vi "Begin.vi"(8 "error in":errorcluster) -> (0 "error out":errorcluster)   [LabVIEW 2023]
doc: "Called before other user functions, this VI is expected to open initial I/O refnums, load in file data, and do all program initialization. Notice that the <B>error out</B> terminal is simply used for data flow. Wiring it to other structures or subVIs ensures that this VI runs first."
uses:
  <vilib>/Rock Robotics/WPI/DriverStation/WPI_DriverStationRobotMode2.ctl
  <vilib>/Rock Robotics/WPI/Joystick/WPI_JoystickDeviceEnum.ctl
  <vilib>/Rock Robotics/WPI/SafetyOutput/WPI_SafetyOutputConfigMenu.ctl
  <vilib>/Rock Robotics/WPI/RobotDrive/WPI_RobotDriveDevRef.ctl
  <vilib>/Rock Robotics/WPI/MotorControl/WPI_MotorControlDeviceRef.ctl
  <vilib>/Rock Robotics/WPI/MotorControl/WPI_MotorControlType.ctl
  <vilib>/Rock Robotics/SystemInterfaces/DIO/FPGA_DIOPWMChannel.ctl
  <vilib>/Rock Robotics/WPI/PWM/WPI_PWMDeadband.ctl
  <vilib>/Rock Robotics/SystemInterfaces/DIO/FPGA_DIOChannel.ctl
  <vilib>/Rock Robotics/WPI/ThirdParty/REV Robotics/REVLib/Typedef/Spark MAX Motor Type.ctl
  <vilib>/Rock Robotics/WPI/ThirdParty/REV Robotics/REVLib/Typedef/Spark MAX Idle Mode.ctl
  Robot Global Data.vi
  <vilib>/Rock Robotics/Network Tables/NT Write String Array.vi
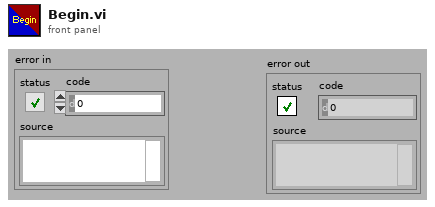
[diagram p1: front panel]
types:
  T1 = typedef "WPI_RobotDriveDevRef.ctl" = cluster{"DevStatus":errorcluster, "Motors[]":T2[], "Square Inputs":bool, "Max Output":dbl}
  T2 = typedef "WPI_MotorControlDeviceRef.ctl" = cluster{"DeviceStatus":errorcluster, "Type":T3, "PWM":cluster{"PWM Channel":T4, "DeadBand":T5}, "CAN":cluster{"Device Number":u8, "SetOutput VI Ref":variant, "GetOutput VI Ref":variant, "Enable VI Ref":variant, "Disable VI Ref":variant, "Data":variant}, "Invert":bool, "DIO PWM":cluster{"PWM \"Enable\" Channel":T4, "DIOChannel":T6, "PWM Rate":dbl}}
  T3 = typedef "WPI_MotorControlType.ctl" = enum16{"PWM", "CAN", "DIO PWM"}
  T4 = typedef "FPGA_DIOPWMChannel.ctl" = enum8{"PWM 0", "PWM 1", "PWM 2", "PWM 3", "PWM 4", "PWM 5", "PWM 6", "PWM 7", "PWM 8", "PWM 9", "PWM MXP 0", "PWM MXP 1", "PWM MXP 2", "PWM MXP 3", "PWM MXP 4", "PWM MXP 5", "PWM MXP 6", "PWM MXP 7", "PWM MXP 8", "PWM MXP 9", "Invalid"}
  T5 = typedef "WPI_PWMDeadband.ctl" = cluster{"Name":string, "maxPositivePwm":i32, "minPositivePwm":i32, "centerPwm":i32, "maxNegativePwm":i32, "minNegativePwm":i32, "angularRange":u16}
  T6 = typedef "FPGA_DIOChannel.ctl" = enum8{"DIO 0", "DIO 1", "DIO 2", "DIO 3", "DIO 4", "DIO 5", "DIO 6", "DIO 7", "DIO 8", "DIO 9", "DIO MXP 0", "DIO MXP 1", "DIO MXP 2", "DIO MXP 3", "DIO MXP 4", "DIO MXP 5", "DIO MXP 6", "DIO MXP 7", "DIO MXP 8", "DIO MXP 9", "DIO MXP 10", "DIO MXP 11", "DIO MXP 12", "DIO MXP 13", "DIO MXP 14", "DIO MXP 15", "SPI Port CS1", "SPI Port CS2", "SPI Port CS3", "SPI Port MISO", "SPI Port MOSI", "Invalid"}
  T7 = typedef "WPI_SafetyOutputConfigMenu.ctl" = enum16{"Enable", "Disable"}
  T8 = typedef "WPI_JoystickDeviceEnum.ctl" = enum16{"USB 0", "USB 1", "USB 2", "USB 3", "USB 4", "USB 5"}
  T9 = typedef "WPI_DriverStationRobotMode2.ctl" = enum16{"Autonomous Disabled", "Autonomous Enabled", "Teleop Disabled", "Teleop Enabled", "Disconnected", "Finish", "Test Disabled", "Test Enabled", "Emergency Stopped"}
  T10 = typedef "Spark MAX Idle Mode.ctl" = enum16{"Coast", "Brake"}
  T11 = typedef "Spark MAX Motor Type.ctl" = enum16{"Brushed", "Brushless"}
  T12 = typedef "WPI_JoystickDevRef.ctl" = cluster{"Device":T8}
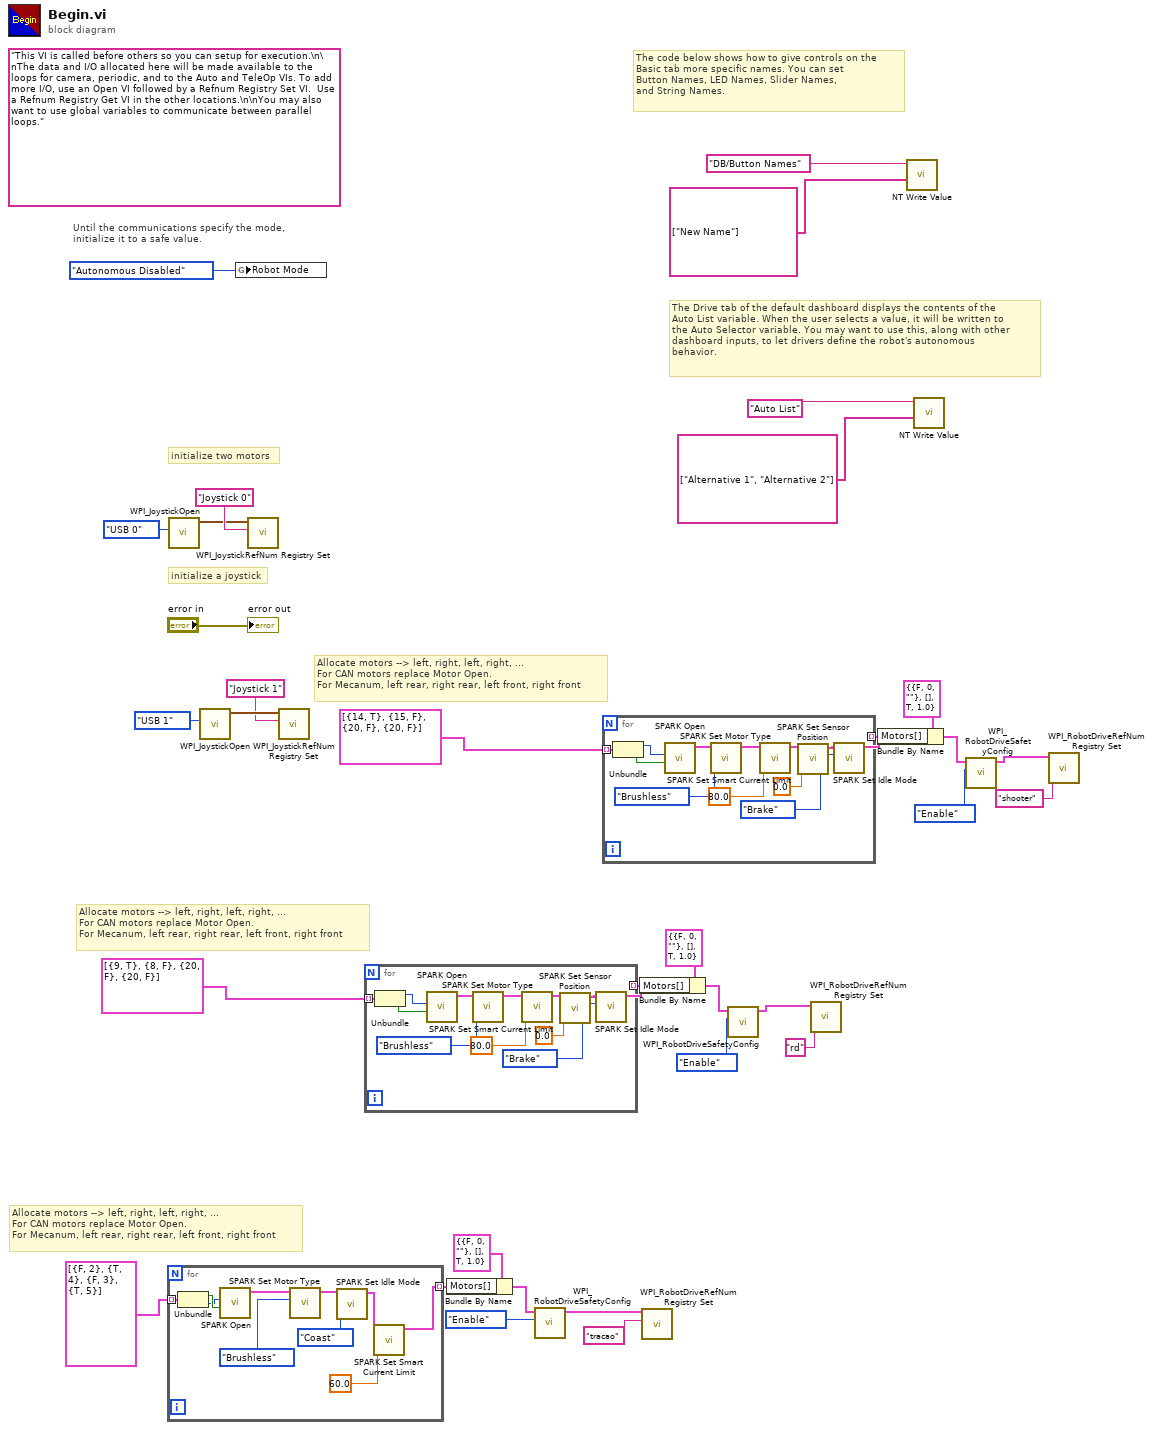
[diagram p0: block diagram]
diagram:
  (unwired) "This VI is called before others so you can setup for execution.\n\nThe data and I/O allocated here will be made available to the loops for camera, periodic, and to the Auto and TeleOp VIs. To add more I/O, use an Open VI followed by a Refnum Registry Set VI.  Use a Refnum Registry Get VI in the other locations.\n\nYou may also want to use global variables to communicate between parallel loops."
  # "Allocate motors --> left, right, left, right, ... \nFor CAN motors replace Motor Open.\nFor Mecanum, left rear, right rear, left front, right front"
  # "Allocate motors --> left, right, left, right, ... \nFor CAN motors replace Motor Open.\nFor Mecanum, left rear, right rear, left front, right front"
  # "Allocate motors --> left, right, left, right, ... \nFor CAN motors replace Motor Open.\nFor Mecanum, left rear, right rear, left front, right front"
  # "The Drive tab of the default dashboard displays the contents of the\nAuto List variable. When the user selects a value, it will be written to\nthe Auto Selector variable. You may want to use this, along with other\ndashboard inputs, to let drivers define the robot's autonomous\nbehavior."
  # "The code below shows how to give controls on the\nBasic tab more specific names. You can set\nButton Names, LED Names, Slider Names,\nand String Names."
  # "initialize a joystick"
  # "Until the communications specify the mode,\ninitialize it to a safe value."
  # "initialize two motors"
  n1 = for {
    tunnel: cluster{"Inverted":bool, "Motor Address":i32}[] [{"Inverted"=FALSE, "Motor Address"=2}, {"Inverted"=TRUE, "Motor Address"=4}, {"Inverted"=FALSE, "Motor Address"=3}, {"Inverted"=TRUE, "Motor Address"=5}] ("Array") -> [w43] mode=indexing
    tunnel: [w35] -> w10 mode=indexing
    n2 = Unbundle(w43) -> ("Inverted"=w42:bool, "Motor Address"=w41:i32)
    n3 = call <vilib>:"SPARK Open.vi"("Invert"=w42, "Device Number"=w41) -> ("MotorControlDeviceRef"=w40:T2)  [unwired: 8 in, 1 out]
    n4 = call <vilib>:"SPARK Set Motor Type.vi"("Motor Type"=Spark_MAX_Motor_Type."Brushless", "MotorControlDevRef"=w40) -> ("MotorControlDeviceRef"=w38:T2)  [unwired: 8 in, 1 out]
    n5 = call <vilib>:"SPARK Set Idle Mode.vi"("Idle Mode"=Spark_MAX_Idle_Mode."Coast", "MotorControlDeviceRef in"=w38) -> ("MotorControlDeviceRef out"=w36:T2)  [unwired: 8 in, 1 out]
    n6 = call <vilib>:"SPARK Set Smart Current Limit.vi"("Primay Current Limit (80A)"=60.0, "MotorControlDeviceRef in"=w36) -> ("MotorControlDeviceRef out"=w35:T2)  [unwired: 8 in, 1 out]
  }
  n7 = call <vilib>:"WPI_JoystickOpen.vi"("JoystickDevice"=WPI_JoystickDeviceEnum."USB 0") -> ("JoystickDevRef"=w31:T12)  [unwired: 10 in]
  n8 = call <vilib>:"WPI_JoystickOpen.vi"("JoystickDevice"=WPI_JoystickDeviceEnum."USB 1") -> ("JoystickDevRef"=w16:T12)  [unwired: 10 in]
  n9 = global write "Robot Global Data.vi" "Robot Mode"(WPI_DriverStationRobotMode2."Autonomous Disabled" ("Robot Mode")) -> ()
  n10 = call <vilib>:"WPI_JoystickRefNum Registry Set.vi"("refnum name"="Joystick 0", "JoystickDevRef"=w31) -> ()  [unwired: 8 in, 2 out]
  n11 = call <vilib>:"WPI_JoystickRefNum Registry Set.vi"("refnum name"="Joystick 1", "JoystickDevRef"=w16) -> ()  [unwired: 8 in, 2 out]
  n12 = for {
    tunnel: cluster{"Motor Address":i32, "Inverted":bool}[] [{"Motor Address"=9, "Inverted"=TRUE}, {"Motor Address"=8, "Inverted"=FALSE}, {"Motor Address"=20, "Inverted"=FALSE}, {"Motor Address"=20, "Inverted"=FALSE}] ("Array") -> [w55] mode=indexing
    tunnel: [w49] -> w20 mode=indexing
    n13 = Unbundle(w55) -> ("Motor Address"=w54:i32, "Inverted"=w53:bool)
    n14 = call <vilib>:"SPARK Open.vi"("Invert"=w53, "Device Number"=w54) -> ("MotorControlDeviceRef"=w52:T2)  [unwired: 8 in, 1 out]
    n15 = call <vilib>:"SPARK Set Motor Type.vi"("Motor Type"=Spark_MAX_Motor_Type."Brushless", "MotorControlDevRef"=w52) -> ("MotorControlDeviceRef"=w48:T2)  [unwired: 8 in, 1 out]
    n16 = call <vilib>:"SPARK Set Smart Current Limit.vi"("Primay Current Limit (80A)"=80.0, "MotorControlDeviceRef in"=w48) -> ("MotorControlDeviceRef out"=w46:T2)  [unwired: 8 in, 1 out]
    n17 = call <vilib>:"SPARK Set Sensor Position.vi"("Position"=0.0, "MotorControlDeviceRef"=w46) -> ("MotorControlDeviceRef"=w45:T2)  [unwired: 8 in, 1 out]
    n18 = call <vilib>:"SPARK Set Idle Mode.vi"("Idle Mode"=Spark_MAX_Idle_Mode."Brake", "MotorControlDeviceRef in"=w45) -> ("MotorControlDeviceRef out"=w49:T2)  [unwired: 8 in, 1 out]
  }
  n19 = Bundle By Name(cluster=T1 {"DevStatus"={"status"=FALSE, "code"=0, "source"=""}, "Motors[]"=[], "Square Inputs"=TRUE, "Max Output"=1.0} ("RobotDriveDevRef"), "Motors[]"=w10) -> (w13:T1)
  n20 = call <vilib>:"WPI_RobotDriveSafetyConfig.vi"("mode"=WPI_SafetyOutputConfigMenu."Enable", "RobotDriveDevRef"=w13) -> ("RobotDriveDevRef"=w9:T1)  [unwired: 2 in, 7 out]
  n21 = for {
    tunnel: cluster{"Motor Address":i32, "Inverted":bool}[] [{"Motor Address"=14, "Inverted"=TRUE}, {"Motor Address"=15, "Inverted"=FALSE}, {"Motor Address"=20, "Inverted"=FALSE}, {"Motor Address"=20, "Inverted"=FALSE}] ("Array") -> [w67] mode=indexing
    tunnel: [w61] -> w5 mode=indexing
    n22 = Unbundle(w67) -> ("Motor Address"=w66:i32, "Inverted"=w65:bool)
    n23 = call <vilib>:"SPARK Open.vi"("Invert"=w65, "Device Number"=w66) -> ("MotorControlDeviceRef"=w64:T2)  [unwired: 8 in, 1 out]
    n24 = call <vilib>:"SPARK Set Motor Type.vi"("Motor Type"=Spark_MAX_Motor_Type."Brushless", "MotorControlDevRef"=w64) -> ("MotorControlDeviceRef"=w60:T2)  [unwired: 8 in, 1 out]
    n25 = call <vilib>:"SPARK Set Smart Current Limit.vi"("Primay Current Limit (80A)"=80.0, "MotorControlDeviceRef in"=w60) -> ("MotorControlDeviceRef out"=w58:T2)  [unwired: 8 in, 1 out]
    n26 = call <vilib>:"SPARK Set Sensor Position.vi"("Position"=0.0, "MotorControlDeviceRef"=w58) -> ("MotorControlDeviceRef"=w57:T2)  [unwired: 8 in, 1 out]
    n27 = call <vilib>:"SPARK Set Idle Mode.vi"("Idle Mode"=Spark_MAX_Idle_Mode."Brake", "MotorControlDeviceRef in"=w57) -> ("MotorControlDeviceRef out"=w61:T2)  [unwired: 8 in, 1 out]
  }
  n28 = Bundle By Name(cluster=T1 {"DevStatus"={"status"=FALSE, "code"=0, "source"=""}, "Motors[]"=[], "Square Inputs"=TRUE, "Max Output"=1.0} ("RobotDriveDevRef"), "Motors[]"=w20) -> (w23:T1)
  n29 = call <vilib>:"WPI_RobotDriveRefNum Registry Set.vi"("refnum name"="tracao", "RobotDriveDevRef"=w9) -> ()  [unwired: 8 in, 2 out]
  n30 = call <vilib>:"WPI_RobotDriveSafetyConfig.vi"("mode"=WPI_SafetyOutputConfigMenu."Enable", "RobotDriveDevRef"=w23) -> ("RobotDriveDevRef"=w19:T1)  [unwired: 2 in, 7 out]
  n31 = call <vilib>:"WPI_RobotDriveRefNum Registry Set.vi"("refnum name"="rd", "RobotDriveDevRef"=w19) -> ()  [unwired: 8 in, 2 out]
  n32 = Bundle By Name(cluster=T1 {"DevStatus"={"status"=FALSE, "code"=0, "source"=""}, "Motors[]"=[], "Square Inputs"=TRUE, "Max Output"=1.0} ("RobotDriveDevRef"), "Motors[]"=w5) -> (w2:T1)
  n33 = call-poly <vilib>:"NT Write Value.vi"("value"=string[] ["New Name"], "name"="DB/Button Names" ("Name")) -> ()  [unwired: 9 in, 1 out]
  n34 = call-poly <vilib>:"NT Write Value.vi"("value"=string[] ["Alternative 1", "Alternative 2"] ("String Array"), "name"="Auto List" ("Name")) -> ()  [unwired: 9 in, 1 out]
  n35 = call <vilib>:"WPI_RobotDriveSafetyConfig.vi"("mode"=WPI_SafetyOutputConfigMenu."Enable", "RobotDriveDevRef"=w2) -> ("RobotDriveDevRef"=w6:T1)  [unwired: 2 in, 7 out]
  n36 = call <vilib>:"WPI_RobotDriveRefNum Registry Set.vi"("refnum name"="shooter", "RobotDriveDevRef"=w6) -> ()  [unwired: 8 in, 2 out]
  "error out" <- "error in"
